vi "Command Listener and OPCUA writer.vi"(6 "port":u16, 9 "Server name":string, 10 "OPCUA Connection in":refnum<k24>, 11 "Stop Reference in":refnum<vi>) -> (0 "error out":errorcluster)   [LabVIEW 2019]
doc: "Multi-client TCP STM listener on supplied port number. Attempts to write received variables to OPCUA server on .NET interface supplied. Will exit when referenced boolean variable goes true."
uses:
  F:/src/HUTCDLSVN/Machine/CDL0100/TagEngine/LVOPCUA.NET/LVOPC.NETInterface/bin/Release/LVOPC.NETInterface.dll
  LVOPCUA.NET/LVOPC.NETInterface/bin/Release/LVOPC.NETInterface.dll
  <vilib>/NI/STM/Connection Manager/TCP/TCP Connection Method.ctl
  <vilib>/NI/STM/SubVIs/MetaDataElement.ctl
  <vilib>/NI/Current Value Table/Type Defs/Single Tag.ctl
  <vilib>/NI/Current Value Table/Type Defs/Data Types.ctl
  <vilib>/Platform/TimedLoop/XDataNode/timing_clust.ctl
  <vilib>/Platform/TimedLoop/XDataNode/nitl_modes.ctl
  <vilib>/Platform/TimedLoop/XDataNode/wakeup.ctl
  <vilib>/NI/STM/TCP/TCP Read Options.ctl
  <vilib>/NI/STM/TCP/Write Meta Data (TCP Ref).vi
  <vilib>/NI/STM/TCP/Write Meta Data (TCP Clst).vi
  <vilib>/NI/STM/TCP/Read Message (TCP).vi
  <vilib>/Platform/TimedLoop/XDataNode/XDataNode.xnode
  <vilib>/NI/STM/NI STM.lvlib
  <vilib>/Platform/TimedLoop/XDataNode/XDNodeRunTimeDep.lvlib
  <vilib>/NI/Current Value Table/Current Value Table.lvlib
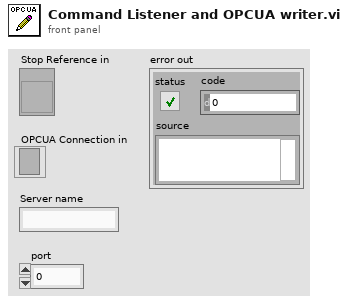
[diagram p1: front panel]
types:
  T1 = typedef "NI STM.lvlib/TCP Connection Method.ctl" = enum16{"Initialize", "Add Connection", "Set Properties", "Get Connection(s)", "Remove Connection", "Remove All Connections", "Get Connection Count"}
  T2 = typedef "Current Value Table.lvlib/Single Tag.ctl" = cluster{"Data Type":T3, "Name":string, "Value":string, "Description":string}
  T3 = typedef "Current Value Table.lvlib/Data Types.ctl" = enum16{"Double", "Single", "I64", "I32", "I16", "I8", "U64", "U32", "U16", "U8", "String", "Boolean", "Array of U8", "Array of U16", "Array of U32", "Array of U64", "Array of I64", "Array of I32", "Array of I16", "Array of I8", "Array of Double", "Array of Single", "Array of Boolean", "Array of String"}
  T4 = typedef "NI STM.lvlib/MetaDataElement.ctl" = string
  T5 = typedef "XDNodeRunTimeDep.lvlib/timing_clust.ctl" = cluster{"Expected End [f-1]":u64, "Actual End [f-1]":u64, "Finished Late? [f-1]":bool, "Expected End [i-1]":u64, "Actual End [i-1]":u64, "Finished Late? [i-1]":bool, "Expected Start [i]":u64, "Actual Start [i]":u64, "Expected Start [f]":u64, "Actual Start [f]":u64, "Source Name":string, "Structure Name":string, "Period":i64, "Deadline":i64, "Offset":i64, "Start":i64, "Priority":i32, "Timeout":i32, "Mode":T6, "Wakeup Reason":T7, "Error":errorcluster, "Source Type":string, "Secondary Source Type":string, "Global End Time":u64, "Global Start Time":u64, "Frame Duration":u64, "Iteration Duration":u64, "Assigned CPU":i32, "I/O Scan Engine Mode":u32}
  T6 = typedef "XDNodeRunTimeDep.lvlib/nitl_modes.ctl" = enum32{"No Change", "Process missed periods, maintain original phase", "Discard missed periods, maintain original phase", "Process missed periods, ignore original phase", "Discard missed periods, ignore original phase"}
  T7 = typedef "XDNodeRunTimeDep.lvlib/wakeup.ctl" = enum32{"Normal", "Aborted", "Asynchronous wakeup", "Timing source error", "Timed loop error", "Timeout"}
  T8 = typedef "NI STM.lvlib/TCP Read Options.ctl" = cluster{"ignore timeout error":bool, "timeout ms (1000)":i32}
  T9 = typedef "NI STM.lvlib/TCP Connection Info.ctl" = cluster{"connection ID":refnum<k5>, "meta data":T4[]}
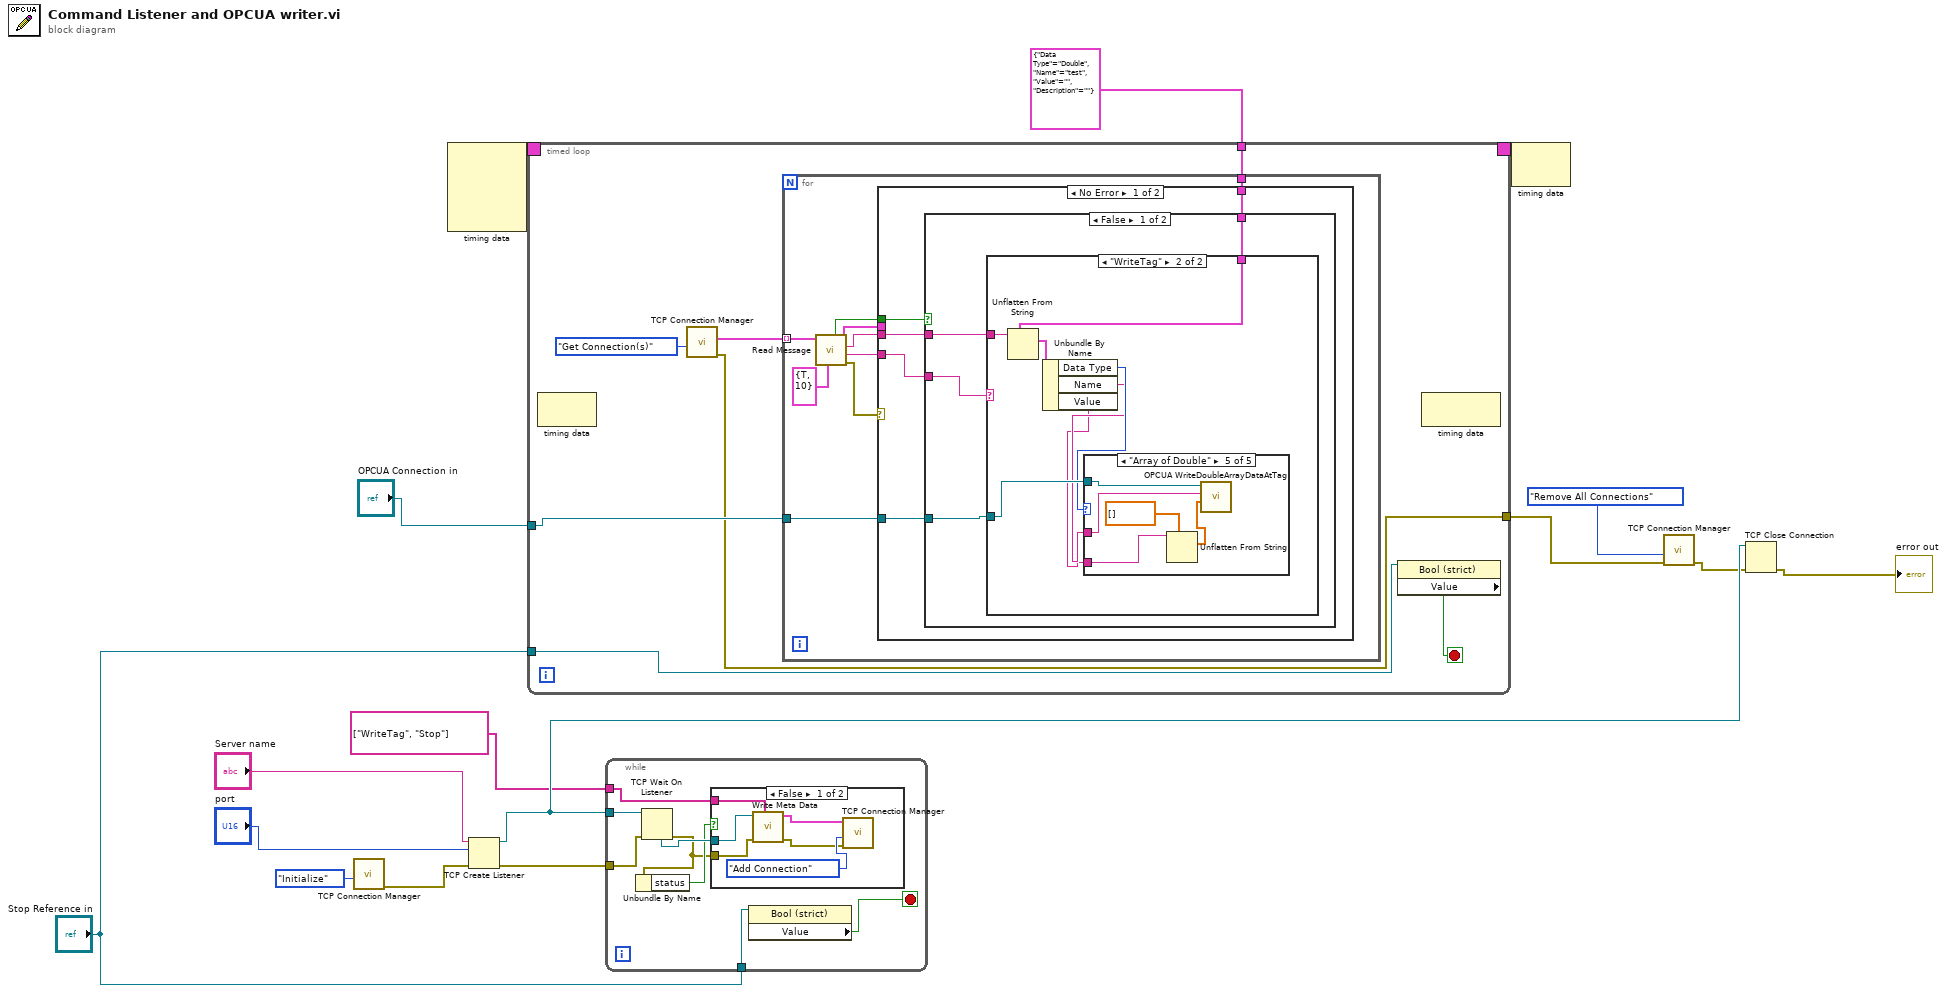
[diagram p0: block diagram]
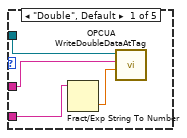
[diagram p3: hidden frame]
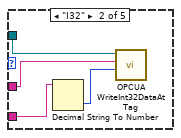
[diagram p4: hidden frame]
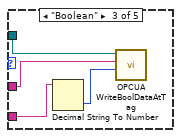
[diagram p5: hidden frame]
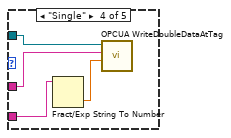
[diagram p6: hidden frame]
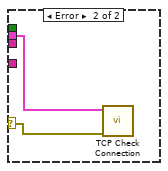
[diagram p8: hidden frame]
diagram:
  n1 = call <vilib>:"TCP Connection Manager.vi"("method"=TCP_Connection_Method."Initialize") -> ("error out"=w3:errorcluster)  [unwired: 5 in, 5 out]
  n2 = node-c288() -> (w16:T5)  [unwired: 4 in]
  n3 = TCP Create Listener(8:w3, 10:"port", 11:"Server name") -> (0:w6:errorcluster, 3:w13:refnum<k5>)  [unwired: 2 in, 1 out]
  n4 = timed-loop {
    timing: w16 -> [_]
    timing-out: [_] -> w15
    tunnel: T2 {"Data Type"=enum."Double", "Name"="test", "Value"="", "Description"=""} ("Tag") -> [w20]
    tunnel: "OPCUA Connection in" -> [w19]
    tunnel: [w18] -> w10
    tunnel: "Stop Reference in" -> [w17]
    stop <- w23 stop-if-true
    n5 = node-c288() -> ()  [unwired: 1 in, 1 out]
    n6 = call <vilib>:"TCP Connection Manager.vi"("method"=TCP_Connection_Method."Get Connection(s)") -> ("error out"=w18:errorcluster, "all connections"=w21:T9[])  [unwired: 5 in, 4 out]
    n7 = for {
      tunnel: w21 -> [w32] mode=indexing
      tunnel: w20 -> [w28]
      tunnel: w19 -> [w26]
      n8 = call-poly <vilib>:"Read Message.vi"("options"=T8 {"ignore timeout error"=TRUE, "timeout ms (1000)"=10}, "connection info in"=w32) -> ("error out"=w31:errorcluster, "name"=w29:T4, "data string"=w27:string, "connection info out"=w24:T9, "timed out?"=w30:bool)  [unwired: 4 in, 1 out]
      n9 = case shown="No Error" w31 {
        selector: w31 -> [_ w71]
        tunnel: w30 -> [w37 _]
        tunnel: w29 -> [w36 _]
        tunnel: w28 -> [w35 _]
        tunnel: w27 -> [w34 _]
        tunnel: w26 -> [w33 _]
        tunnel: w24 -> [_ w70]
        frame No Error {
          n10 = case shown="False" w37 {
            tunnel: w36 -> [w41 _]
            tunnel: w35 -> [w40 _]
            tunnel: w34 -> [w39 _]
            tunnel: w33 -> [w38 _]
            frame False {
              n11 = case shown="\"WriteTag\"" w41 {
                tunnel: w40 -> [_ w47]
                tunnel: w39 -> [_ w48]
                tunnel: w38 -> [_ w45]
                frame "False", Default {
                }
                frame "WriteTag" {
                  n12 = Unflatten From String(type=w47, binary string=w48) -> (value=w46:T2)  [unwired: 3 in, 2 out]
                  n13 = Unbundle By Name(w46) -> ("Data Type"=w44:T3, "Name"=w43:string, "Value"=w42:string)
                  n14 = case shown="\"Array of Double\"" w44 {
                    tunnel: w45 -> [w52 w56 w60 w64 w69]
                    tunnel: w43 -> [w51 w55 w59 w63 w68]
                    tunnel: w42 -> [w49 w54 w58 w61 w67]
                    frame "Double", Default {
                      n15 = Fract/Exp String To Number(string=w49) -> (number=w50:dbl)  [unwired: 3 in, 1 out]
                      n16 = call "OPCUA WriteDoubleDataAtTag.vi"("value"=w50, "tag"=w51, "reference"=w52) -> ()  [unwired: 6 in, 3 out]
                    }
                    frame "I32" {
                      n17 = Decimal String To Number(string=w54) -> (number=w53:i32)  [unwired: 2 in, 1 out]
                      n18 = call "OPCUA WriteInt32DataAtTag.vi"("value"=w53, "tag"=w55, "reference"=w56) -> ()  [unwired: 6 in, 3 out]
                    }
                    frame "Boolean" {
                      n19 = Decimal String To Number(string=w58) -> (number=w57:i32)  [unwired: 2 in, 1 out]
                      n20 = call "OPCUA WriteBoolDataAtTag.vi"("value"=w57, "tag"=w59, "reference"=w60) -> ()  [unwired: 6 in, 3 out]
                    }
                    frame "Single" {
                      n21 = Fract/Exp String To Number(string=w61) -> (number=w62:dbl)  [unwired: 3 in, 1 out]
                      n22 = call "OPCUA WriteDoubleDataAtTag.vi"("value"=w62, "tag"=w63, "reference"=w64) -> ()  [unwired: 6 in, 3 out]
                    }
                    frame "Array of Double" {
                      n23 = Unflatten From String(type=dbl[] [], binary string=w67) -> (value=w65:dbl[])  [unwired: 3 in, 2 out]
                      n24 = call "OPCUA WriteDoubleArrayDataAtTag.vi"("val"=w65, "tag"=w68, "reference"=w69) -> ()  [unwired: 6 in, 3 out]
                    }
                  }
                }
              }
            }
            frame True {
            }
          }
        }
        frame Error {
          n25 = call <vilib>:"TCP Check Connection.vi"("error in"=w71, "connection in"=w70) -> ()  [unwired: 7 in, 3 out]
        }
      }
    }
    n26 = property class="Bool (strict)"(reference=w17) -> ("Value"=w23:bool)  [unwired: 1 in, 2 out]
    n27 = node-c288() -> ()  [unwired: 1 in, 1 out]
  }
  n28 = while {
    tunnel: w13 -> [w81]
    tunnel: w6 -> [w80]
    tunnel: T4[] ["WriteTag", "Stop"] ("meta data") -> [w77]
    tunnel: "Stop Reference in" -> [w74]
    stop <- w76 stop-if-true
    n29 = TCP Wait On Listener(8:w80, 11:w81) -> (0:w75:errorcluster, 4:w79:refnum<k5>)  [unwired: 2 in, 3 out]
    n30 = Unbundle By Name(w75) -> ("status"=w78:bool)
    n31 = case shown="False" w78 {
      tunnel: w79 -> [w85 _]
      tunnel: w77 -> [w84 _]
      tunnel: w75 -> [w82 _]
      frame False {
        n32 = call-poly <vilib>:"Write Meta Data.vi"("meta data"=w84, "error in"=w82, "connection ID"=w85) -> ("error out"=w83:errorcluster, "connection info out"=w87:T9)  [unwired: 2 in, 5 out]
        n33 = call <vilib>:"TCP Connection Manager.vi"("error in"=w83, "method"=TCP_Connection_Method."Add Connection", "connection in"=w87) -> ()  [unwired: 3 in, 6 out]
      }
      frame True {
      }
    }
    n34 = property class="Bool (strict)"(reference=w74) -> ("Value"=w76:bool)  [unwired: 1 in, 2 out]
  }
  n35 = node-c288(w15) -> ()  [unwired: 1 out]
  n36 = call <vilib>:"TCP Connection Manager.vi"("error in"=w10, "method"=TCP_Connection_Method."Remove All Connections") -> ("error out"=w12:errorcluster)  [unwired: 4 in, 5 out]
  n37 = TCP Close Connection(connection ID=w13, error in (no error)=w12) -> (error out=→"error out":errorcluster)  [unwired: 1 in, 1 out]
